vi "Renishaw-XL80_GetMatCompFactor.vi"(8 "error in (no error)":errorcluster, 11 "Renishaw-XL80_EMU in":refnum<class "Renishaw-XL80_EMU.lvclass">) -> (0 "error out":errorcluster, 2 "MatCompFactor":dbl, 3 "Renishaw-XL80_EMU out":refnum<class "Renishaw-XL80_EMU.lvclass">)   [LabVIEW 2024, in "Renishaw-XL80_EMU.lvclass"]
doc: "Reading this property retrieves the current material compensation factor.\n\nDefinition\nHRESULTget_MatCompFactor( [out, retval] double* pVal);\nParameters\npVal\nA variable that will be set to the current material compensation factor.\n\nComments\nReading this property will always retrieve the current material compensation factor. The material compensation factor is a factor which when multiplied by the raw laser measurement will compensate the reading for thermal growth of the material, thereby estimating the reading that would be obtained if the material temperature had been 20°C. Note that MatCompFactor is a value very close to 1.00. For example if the expansion coefficient is set to 10ppm/°C and the current material temperature is 25°C then MatCompFactor will be 0.9999\n\nThe property will normally return an HRESULT of S_OK. However, it will return E_POINTER if the client supplies a null pointer for pVal."
uses:
  Renishaw-XL80_EMU.lvclass
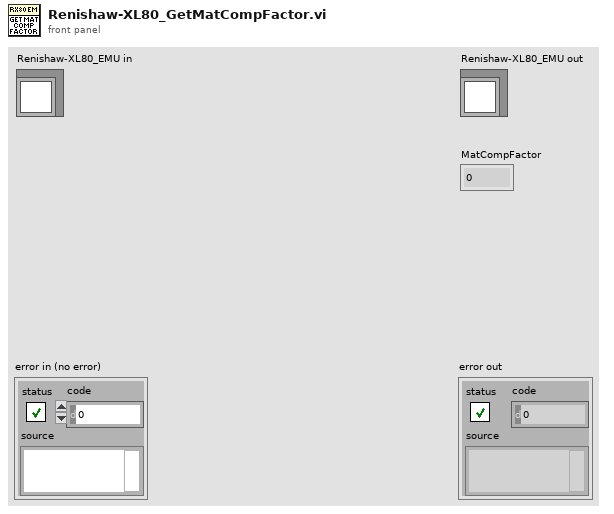
[diagram p1: front panel]
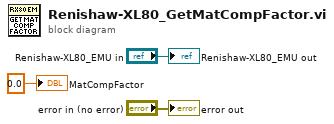
[diagram p0: block diagram]
diagram:
  "error out" <- "error in (no error)"
  "Renishaw-XL80_EMU out" <- "Renishaw-XL80_EMU in"
  "MatCompFactor" <- 0.0 ("MatCompFactor")
